vi "median_filter.vi"(1 "X":fxp<+/-,24,3> format="%.22g") -> (0 "Y":fxp<+/-,24,3> format="%.22g")   [LabVIEW 2018]
uses:
  <vilib>/rvi/Emulation/niFpgaGetClockAttributes.vi
  <vilib>/rvi/Emulation/niFpgaSctlEmulationGetInTimedLoop.vi
  <vilib>/rvi/Emulation/niFpgaEmulationReportErrorSimple.vi
  <vilib>/rvi/DataTransferAndStorage/Container/Common/niFpgaContainerGetUniqueNameForEmu.vi
  <vilib>/rvi/DataTransferAndStorage/Container/Common/niFpgaContainerSetEmuInfo.vi
  <vilib>/rvi/eio/common/nirviEmuReportErrorAndStop.vi
  <vilib>/rvi/DataTransferAndStorage/Container/Common/niFpgaContainerExecOnDevCompGetState.vi
  <vilib>/rvi/Emulation/niFpgaEmulationIsFPGAContextNoSignature.vi
  <vilib>/rvi/Emulation/niFpgaProcessEmulError.vi
  <vilib>/rvi/errors/nirviReportUnexpectedCaseInternalError (U32).vi
  <vilib>/rvi/Memory/Memory_Emulation/niFpgaMemoryEmulationCacheClearOnFirstRun.vi
  <vilib>/rvi/Memory/Memory_Emulation/nirvimemoryEmulationManagerCache_MakeExclusive.vi
  <vilib>/rvi/Memory/Memory_Emulation/niFpgaMemoryEmulationValidateCache.vi
  <vilib>/rvi/Memory/Memory_Emulation/nirvimemoryEmulationManagerCache_InsertValue.vi
  <vilib>/Utility/error.llb/Clear Errors.vi
  <vilib>/rvi/Memory/Memory_Emulation/nirvimemoryEmulationManagerCache_ReleaseExclusive.vi
  <vilib>/rvi/Memory/Memory_Emulation/nirvimemoryEmulationManagerCache_GetValue.vi
  <vilib>/rvi/Memory/Memory_Emulation/nirvimemoryEmulationManagerCache_SetValue.vi
  <vilib>/rvi/Emulation/niFpgaSctlEmulationResourceMgr.vi
  <vilib>/rvi/Emulation/niFpgaCriticalErrorInLSC.vi
  <vilib>/rvi/LocalResourceManager/LocalResourceManager.xnode
  <vilib>/rvi/DataTransferAndStorage/Container/XNode/niFpgaContainer.xnode
  <vilib>/rvi/Memory/Memory_Emulation/niFpgaMemoryEmulationRefIn.vi
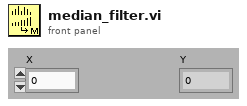
[diagram p1: front panel]
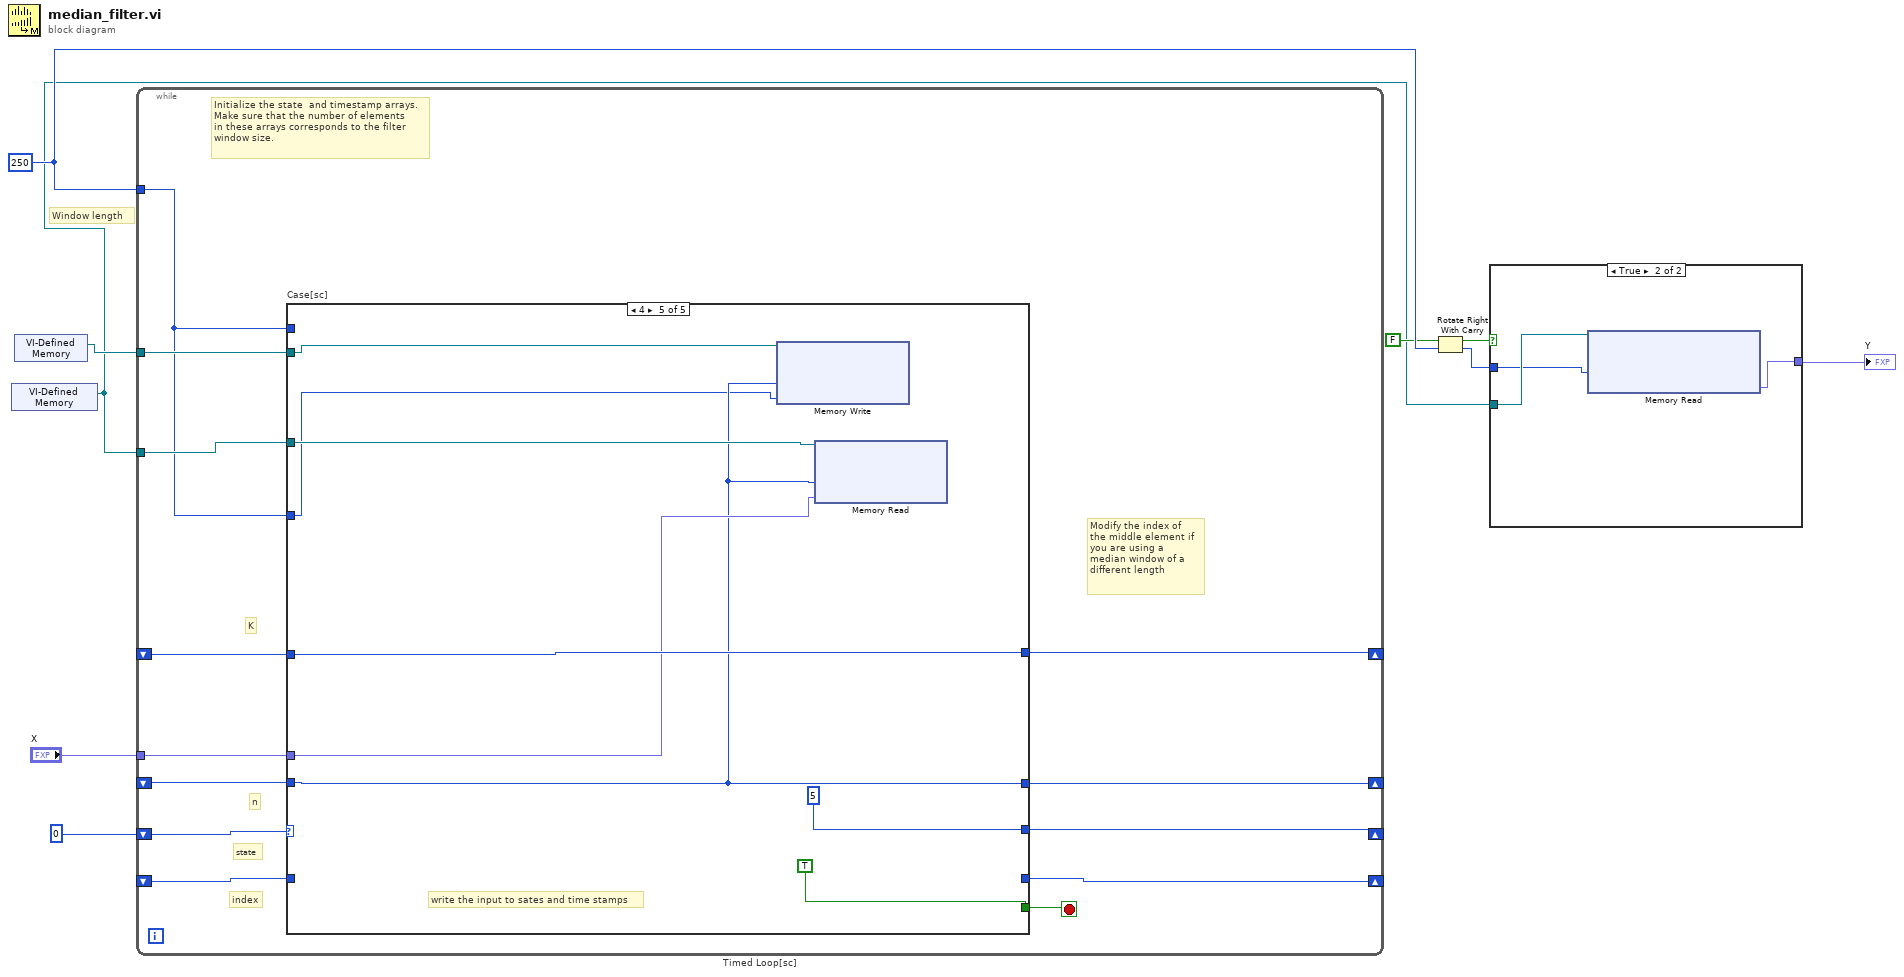
[diagram p0: block diagram]
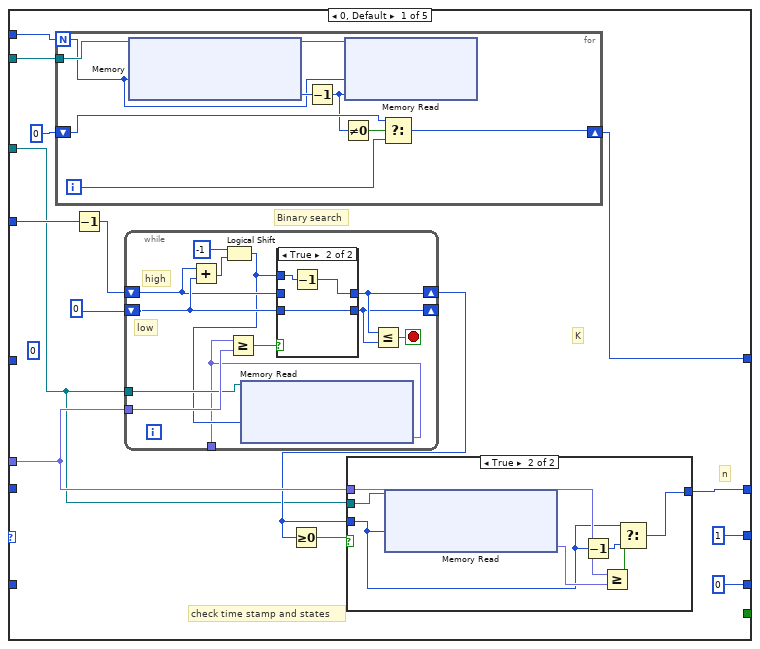
[diagram p2: hidden frame]
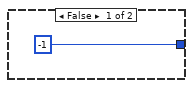
[diagram p3: hidden frame]
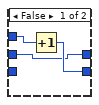
[diagram p4: hidden frame]
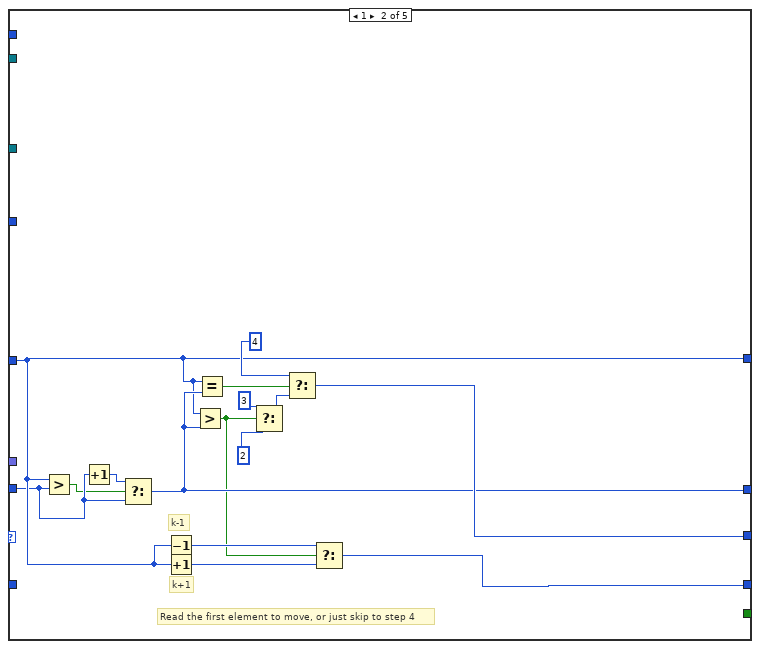
[diagram p5: hidden frame]
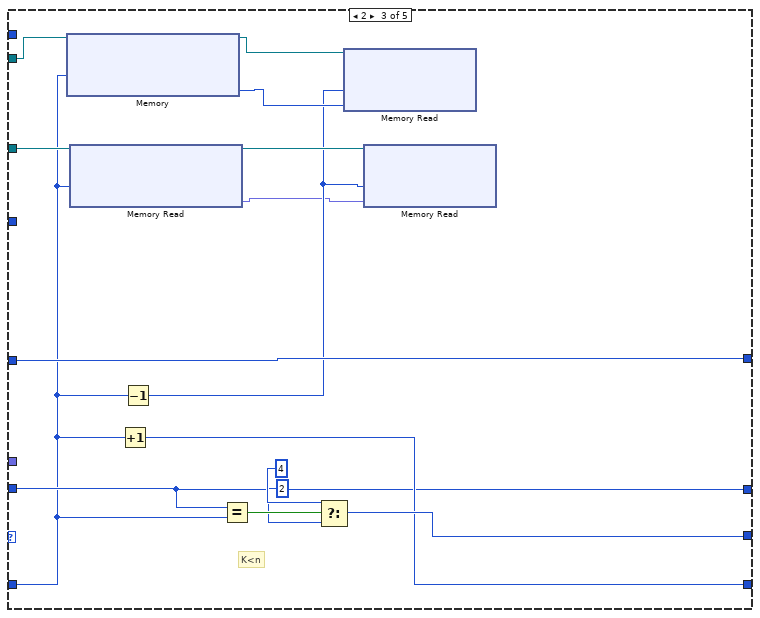
[diagram p6: hidden frame]
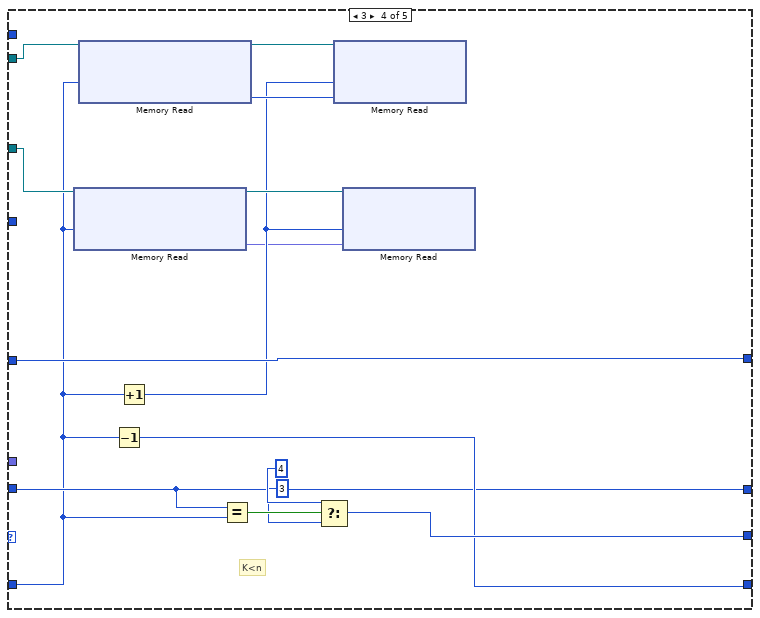
[diagram p7: hidden frame]
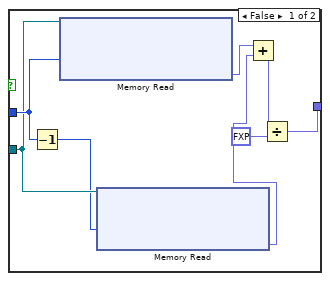
[diagram p8: hidden frame]
diagram:
  w7 = 250 ("Window size")
  # "Window length"
  n1 = xnode "VI-Defined Memory"() -> ("Memory Out"=w1:refnum<k21>)
  n2 = xnode "VI-Defined Memory"() -> ("Memory Out"=w2:refnum<k21>)
  n3 = while "Timed Loop[sc]" {
    tunnel: "X" -> [w22]
    shift-right: [w11] -> _
    shift-left: _ -> [w21]
    shift-right: [w19] -> _
    shift-left: u8 0 ("f") -> [w20]
    shift-right: [w17] -> _
    shift-left: _ -> [w18]
    tunnel: w7 -> [w10]
    shift-right: [w15] -> _
    shift-left: _ -> [w14]
    tunnel: w2 -> [w13]
    tunnel: w1 -> [w12]
    stop <- w16 stop-if-true
    # "Initialize the state  and timestamp arrays.\nMake sure that the number of elements \nin these arrays corresponds to the filter\nwindow size."
    # "Modify the index of \nthe middle element if\nyou are using a\nmedian window of a \ndifferent length"
    # "state"
    # "index"
    # "n"
    # "K"
    n4 = case "Case[sc]" shown="4" w20 {
      tunnel: [0 w74 w96 w111 _] -> w17
      tunnel: [u8 1 ("f") w81 w98 w113 u8 5] -> w19
      tunnel: w22 -> [w32 _ _ _ w119]
      tunnel: [w24 w76 w97 w112 w123] -> w11
      tunnel: w21 -> [_ w76 w97 w112 w123]
      tunnel: [w31 w78 w95 w110 w118] -> w15
      tunnel: w18 -> [_ _ w90 w105 _]
      tunnel: [_ _ _ _ TRUE] -> w16
      tunnel: w14 -> [_ w75 w95 w110 w118]
      tunnel: w13 -> [w28 _ w94 w109 w121]
      tunnel: w10 -> [w26 _ _ _ w117]
      tunnel: w12 -> [w25 _ w91 w106 w120]
      tunnel: w10 -> [w23 _ _ _ _]
      frame 0, Default {
        (unwired) 0 ("index")
        # "Binary search"
        # "n"
        # "K"
        # "check time stamp and states"
        n5 = for {
          N: w23 -> [w67]
          tunnel: w28 -> [w71]
          shift-right: [w63] -> w24
          shift-left: i16 0 ("f") -> [w65]
          i -> [w66]
          n6 = xnode "Memory"("Address"=w67, "Memory In"=w71) -> ("Data"=w70:i16, "Memory Out"=w68:refnum<k21>)
          n7 = Decrement(x=w70) -> (x-1=w64:i16)
          n8 = Not Equal To 0?(x=w64) -> (x != 0?=w69:bool)
          n9 = xnode "Memory Read"("Address"=w67, "Data"=w64, "Memory In"=w68) -> ()  [unwired: 1 out]
          n10 = Select(t=w65, s=w69, f=w66) -> (s? t:f=w63:i32)
        }
        n11 = Decrement(x=w26) -> (x-1=w33:i16)
        n12 = while {
          shift-right: [w50] -> w30
          shift-left: w33 -> [w51]
          tunnel: w32 -> [w53]
          shift-right: [w49] -> _
          shift-left: i16 0 -> [w52]
          tunnel: [w45] -> _
          tunnel: w25 -> [w47]
          stop <- w48 stop-if-true
          # "low"
          # "high"
          n13 = Add(x=w51, y=w52) -> (x+y=w56:i16)
          n14 = Logical Shift(y=i16 -1, x=w56) -> (x << y=w46:i16)
          n15 = xnode "Memory Read"("Address"=w46, "Memory In"=w47) -> ("Data"=w45:fxp<+/-,24,5>)  [unwired: 1 out]
          n16 = Greater Or Equal?(x=w45, y=w53) -> (x >= y?=w54:bool)
          n17 = case shown="True" w54 {
            tunnel: w46 -> [w59 w62]
            tunnel: w52 -> [_ w61]
            tunnel: [w58 w61] -> w49
            tunnel: w51 -> [w57 _]
            tunnel: [w57 w60] -> w50
            frame False {
              n18 = Increment(x=w59) -> (x+1=w58:i16)
            }
            frame True {
              n19 = Decrement(x=w62) -> (x-1=w60:i16)
            }
          }
          n20 = Less Or Equal?(x=w50, y=w49) -> (x <= y?=w48:bool)
        }
        n21 = Greater Or Equal To 0?(x=w30) -> (x >= 0?=w29:bool)
        n22 = case shown="True" w29 {
          tunnel: w32 -> [_ w44]
          tunnel: [i16 -1 w41] -> w31
          tunnel: w30 -> [_ w38]
          tunnel: w25 -> [_ w40]
          frame False {
          }
          frame True {
            n23 = xnode "Memory Read"("Address"=w38, "Memory In"=w40) -> ("Data"=w39:fxp<+/-,24,5>)  [unwired: 1 out]
            n24 = Decrement(x=w38) -> (x-1=w42:i16)
            n25 = Greater Or Equal?(x=w44, y=w39) -> (x >= y?=w43:bool)
            n26 = Select(t=w38, s=w43, f=w42) -> (s? t:f=w41:i16)
          }
        }
      }
      frame 1 {
        # "k+1"
        # "k-1"
        # "Read the first element to move, or just skip to step 4"
        n27 = Greater?(x=w76, y=w75) -> (0:w72:bool)
        n28 = Increment(x=w75) -> (x+1=w73:i16)
        n29 = Select(t=w73, s=w72, f=w75) -> (s? t:f=w78:i16)
        n30 = Decrement(x=w76) -> (x-1=w79:i16)
        n31 = Increment(x=w76) -> (x+1=w80:i16)
        n32 = Greater?(x=w76, y=w78) -> (0:w77:bool)
        n33 = Equal?(x=w76, y=w78) -> (x = y?=w86:bool)
        n34 = Select(t=u8 3, s=w77, f=u8 2) -> (s? t:f=w82:u8)
        n35 = Select(t=u8 4, s=w86, f=w82) -> (s? t:f=w81:u8)
        n36 = Select(t=w79, s=w77, f=w80) -> (s? t:f=w74:i16)
      }
      frame 2 {
        # "K<n"
        n37 = xnode "Memory"("Address"=w90, "Memory In"=w94) -> ("Data"=w92:i16, "Memory Out"=w93:refnum<k21>)
        n38 = xnode "Memory Read"("Address"=w90, "Memory In"=w91) -> ("Data"=w87:fxp<+/-,24,5>, "Memory Out"=w89:refnum<k21>)
        n39 = Increment(x=w90) -> (x+1=w96:i16)
        n40 = Decrement(x=w90) -> (x-1=w88:i16)
        n41 = Equal?(x=w95, y=w90) -> (x = y?=w101:bool)
        n42 = Select(t=u8 4, s=w101, f=u8 2) -> (s? t:f=w98:u8)
        n43 = xnode "Memory Read"("Address"=w88, "Data"=w92, "Memory In"=w93) -> ()  [unwired: 1 out]
        n44 = xnode "Memory Read"("Address"=w88, "Data"=w87, "Memory In"=w89) -> ()  [unwired: 1 out]
      }
      frame 3 {
        # "K<n"
        n45 = xnode "Memory Read"("Address"=w105, "Memory In"=w106) -> ("Data"=w102:fxp<+/-,24,5>, "Memory Out"=w104:refnum<k21>)
        n46 = xnode "Memory Read"("Address"=w105, "Memory In"=w109) -> ("Data"=w107:i16, "Memory Out"=w108:refnum<k21>)
        n47 = Decrement(x=w105) -> (x-1=w111:i16)
        n48 = Increment(x=w105) -> (x+1=w103:i16)
        n49 = Equal?(x=w110, y=w105) -> (x = y?=w116:bool)
        n50 = Select(t=u8 4, s=w116, f=u8 3) -> (s? t:f=w113:u8)
        n51 = xnode "Memory Read"("Address"=w103, "Data"=w107, "Memory In"=w108) -> ()  [unwired: 1 out]
        n52 = xnode "Memory Read"("Address"=w103, "Data"=w102, "Memory In"=w104) -> ()  [unwired: 1 out]
      }
      frame 4 {
        # "write the input to sates and time stamps"
        n53 = xnode "Memory Write"("Address"=w118, "Data"=w117, "Memory In"=w121) -> ()  [unwired: 1 out]
        n54 = xnode "Memory Read"("Address"=w118, "Data"=w119, "Memory In"=w120) -> ()  [unwired: 1 out]
      }
    }
  }
  n55 = Rotate Right With Carry(2:w7, 3:FALSE ("carry")) -> (0:w4:i32, 1:w6:bool)
  n56 = case shown="True" w6 {
    tunnel: [w132 w133] -> w5
    tunnel: w4 -> [w129 w134]
    tunnel: w1 -> [w128 w135]
    frame False {
      n57 = Decrement(x=w129) -> (x-1=w127:i32)
      n58 = xnode "Memory Read"("Address"=w129, "Memory In"=w128) -> ("Data"=w126:fxp<+/-,24,5>)  [unwired: 1 out]
      n59 = xnode "Memory Read"("Address"=w127, "Memory In"=w128) -> ("Data"=w125:fxp<+/-,24,5>)  [unwired: 1 out]
      n60 = Add(x=w126, y=w125) -> (x+y=w131:fxp<+/-,25,6>)
      n61 = Divide(x=w131, y=fxp<+/-,25,4> 2.0) -> (x/y=w132:fxp<+/-,51,28>)
    }
    frame True {
      n62 = xnode "Memory Read"("Address"=w134, "Memory In"=w135) -> ("Data"=w133:fxp<+/-,24,5>)  [unwired: 1 out]
    }
  }
  "Y" <- w5
